vi "Intake Control.vi"(11 "Intake Encoder Angle":dbl=0.25) -> (3 "Intake Motor Power":dbl)   [LabVIEW 2017]
uses:
  Global Variables.vi
panel:
  in  "Range":dbl=60.0
  in  "Torque Compensation Power":dbl=0.2
  in  "Takeoff Power":dbl=0.7999999999999999
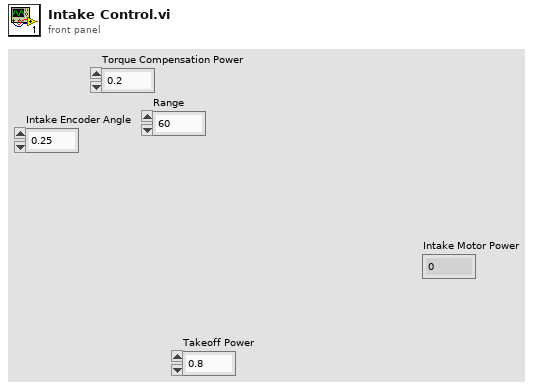
[diagram p1: front panel]
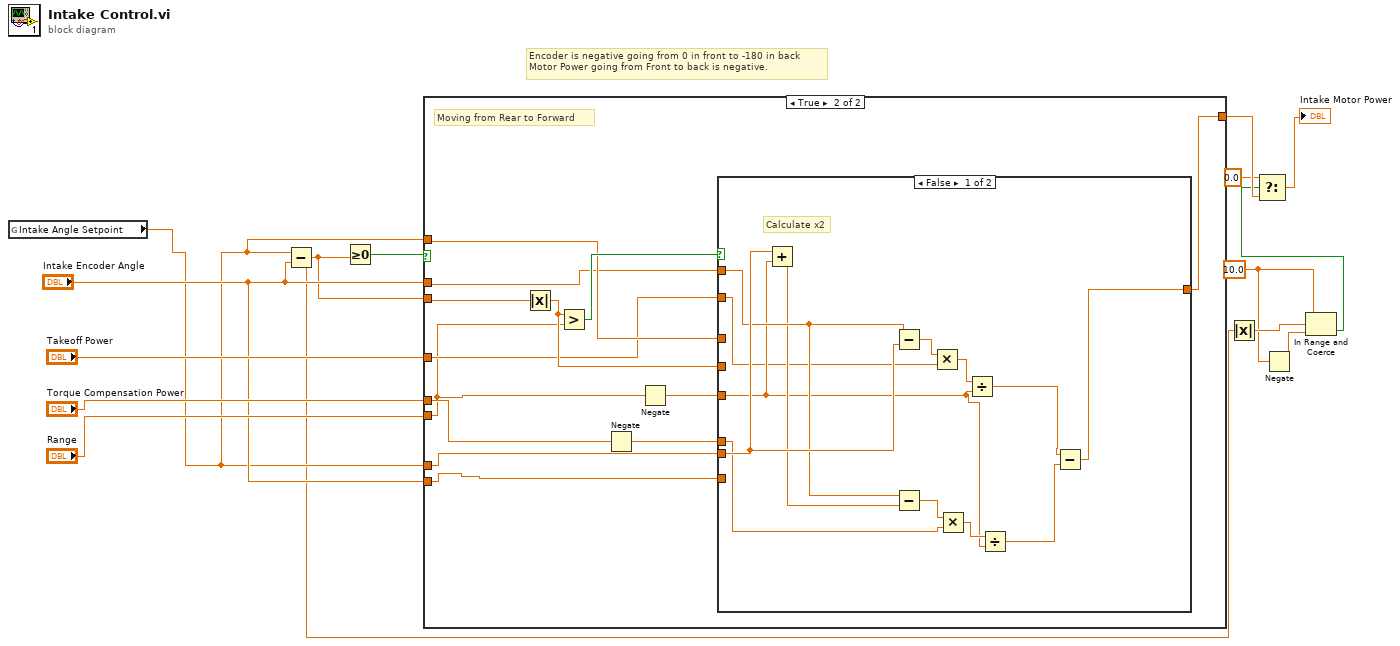
[diagram p0: block diagram]
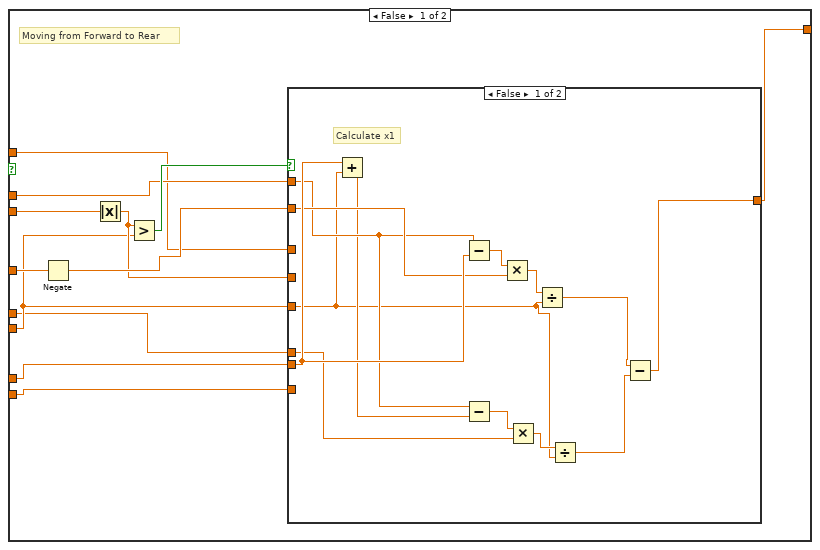
[diagram p2: hidden frame]
diagram:
  w4 = 10.0 ("upper limit")
  # "Encoder is negative going from 0 in front to -180 in back\nMotor Power going from Front to back is negative."
  n1 = global read "Global Variables.vi" "Intake Angle Setpoint"() -> (w9:dbl)
  n2 = Subtract(x=w9, y="Intake Encoder Angle") -> (x-y=w6:dbl)
  n3 = Greater Or Equal To 0?(x=w6) -> (x >= 0?=w14:bool)
  n4 = case shown="True" w14 {
    tunnel: "Takeoff Power" -> [w24 w48]
    tunnel: "Torque Compensation Power" -> [w17 w47]
    tunnel: "Range" -> [w20 w46]
    tunnel: w6 -> [w26 w49]
    tunnel: [w23 w43] -> w8
    tunnel: "Intake Encoder Angle" -> [w19 w50]
    tunnel: w9 -> [w18 w51]
    tunnel: "Intake Encoder Angle" -> [w16 w44]
    tunnel: w9 -> [w15 w45]
    frame False {
      # "Moving from Forward to Rear"
      n5 = Negate(x=w24) -> (-x=w22:dbl)
      n6 = Absolute Value(x=w26) -> (abs(x)=w21:dbl)
      n7 = Greater?(x=w21, y=w20) -> (0:w25:bool)
      n8 = case shown="False" w25 {
        tunnel: w22 -> [w37 w40]
        tunnel: [w27 w40] -> w23
        tunnel: w21 -> [_ _]
        tunnel: w20 -> [w30 _]
        tunnel: w19 -> [w35 _]
        tunnel: w18 -> [_ _]
        tunnel: w17 -> [w32 _]
        tunnel: w16 -> [_ _]
        tunnel: w15 -> [w39 _]
        frame False {
          # "Calculate x1"
          n9 = Add(x=w39, y=w30) -> (x+y=w34:dbl)
          n10 = Subtract(x=w35, y=w39) -> (x-y=w38:dbl)
          n11 = Subtract(x=w35, y=w34) -> (x-y=w33:dbl)
          n12 = Multiply(x=w38, y=w37) -> (x*y=w36:dbl)
          n13 = Multiply(x=w33, y=w32) -> (x*y=w31:dbl)
          n14 = Divide(x=w36, y=w30) -> (x/y=w29:dbl)
          n15 = Divide(x=w31, y=w30) -> (x/y=w28:dbl)
          n16 = Subtract(x=w29, y=w28) -> (x-y=w27:dbl)
        }
        frame True {
        }
      }
    }
    frame True {
      # "Moving from Rear to Forward"
      n17 = Absolute Value(x=w49) -> (abs(x)=w52:dbl)
      n18 = Greater?(x=w52, y=w46) -> (0:w53:bool)
      n19 = Negate(x=w47) -> (-x=w42:dbl)
      n20 = Negate(x=w46) -> (-x=w41:dbl)
      n21 = case shown="False" w53 {
        tunnel: w48 -> [w55 w67]
        tunnel: [w56 w67] -> w43
        tunnel: w52 -> [_ _]
        tunnel: w41 -> [w59 _]
        tunnel: w50 -> [w63 _]
        tunnel: w51 -> [_ _]
        tunnel: w42 -> [w54 _]
        tunnel: w44 -> [_ _]
        tunnel: w45 -> [w66 _]
        frame False {
          # "Calculate x2"
          n22 = Add(x=w66, y=w59) -> (x+y=w62:dbl)
          n23 = Subtract(x=w63, y=w66) -> (x-y=w65:dbl)
          n24 = Subtract(x=w63, y=w62) -> (x-y=w61:dbl)
          n25 = Multiply(x=w65, y=w55) -> (x*y=w64:dbl)
          n26 = Multiply(x=w61, y=w54) -> (x*y=w60:dbl)
          n27 = Divide(x=w64, y=w59) -> (x/y=w58:dbl)
          n28 = Divide(x=w60, y=w59) -> (x/y=w57:dbl)
          n29 = Subtract(x=w58, y=w57) -> (x-y=w56:dbl)
        }
        frame True {
        }
      }
    }
  }
  n30 = Absolute Value(x=w6) -> (abs(x)=w5:dbl)
  n31 = Negate(x=w4) -> (-x=w3:dbl)
  n32 = In Range and Coerce(upper limit=w4, x=w5, lower limit=w3) -> (In Range?=w2:bool)  [unwired: 1 out]
  n33 = Select(t=0.0, s=w2, f=w8) -> (s? t:f=→"Intake Motor Power":dbl)
